vi "Write Sensor Attributes.vi"(9 "New":T1, 11 "Sensor DAO Class in":refnum<class "Sensor DAO Class.lvclass">) -> (3 "Sensor DAO Class out":refnum<class "Sensor DAO Class.lvclass">)   [LabVIEW 2013]
uses:
  Sensor DAO Class.lvclass
  XControls/Sensor Metadata.ctl
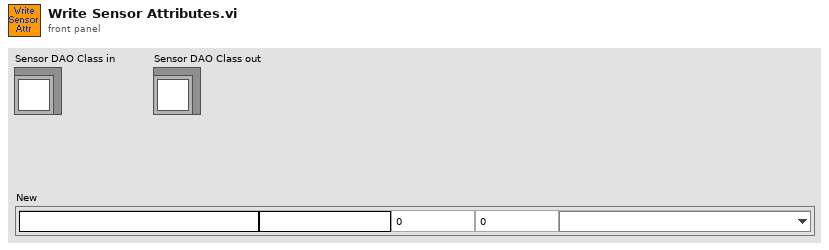
[diagram p1: front panel]
types:
  T1 = typedef "Sensor Metadata.ctl" = cluster{"Name":string, "Units":string, "Multiplier":dbl, "Excitation":u16, "Sensitivity":dbl}
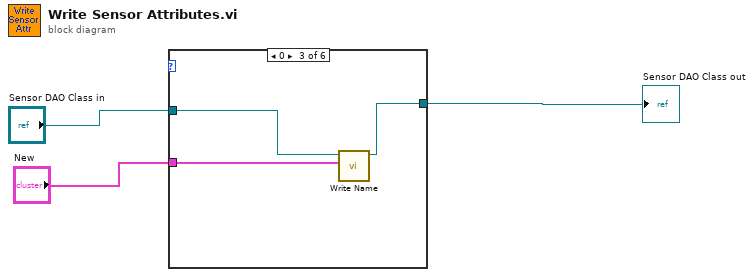
[diagram p0: block diagram]
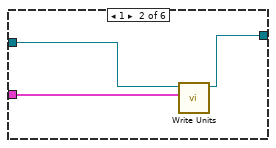
[diagram p3: hidden frame]
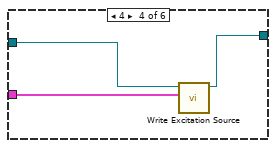
[diagram p4: hidden frame]
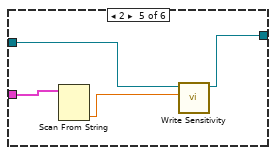
[diagram p5: hidden frame]
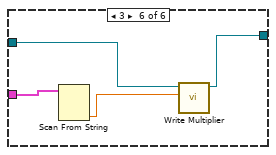
[diagram p6: hidden frame]
diagram:
  n1 = case shown="0" w1 {
    tunnel: "New" -> [_ w8 w11 w14 w18 w22]
    tunnel: "Sensor DAO Class in" -> [w5 w7 w10 w13 w17 w21]
    tunnel: [w5 w6 w9 w12 w16 w20] -> w4
    frame -1, Default {
    }
    frame 1 {
      n2 = call "Write Units.vi"("Units"=w8, "Sensor DAO Class in"=w7) -> ("Sensor DAO Class out"=w6:refnum<class "Sensor DAO Class.lvclass">)  [unwired: 8 in, 1 out]
    }
    frame 0 {
      n3 = call "Write Name.vi"("Name"=w11, "Sensor DAO Class in"=w10) -> ("Sensor DAO Class out"=w9:refnum<class "Sensor DAO Class.lvclass">)  [unwired: 8 in, 1 out]
    }
    frame 4 {
      n4 = call "Write Excitation Source.vi"("Excitation Source"=w14, "Sensor DAO Class in"=w13) -> ("Sensor DAO Class out"=w12:refnum<class "Sensor DAO Class.lvclass">)  [unwired: 8 in, 1 out]
    }
    frame 2 {
      n5 = Scan From String(input string=w18) -> (output 1=w15:dbl)  [unwired: 4 in, 3 out]
      n6 = call "Write Sensitivity.vi"("Sensitivity"=w15, "Sensor DAO Class in"=w17) -> ("Sensor DAO Class out"=w16:refnum<class "Sensor DAO Class.lvclass">)  [unwired: 8 in, 1 out]
    }
    frame 3 {
      n7 = Scan From String(input string=w22) -> (output 1=w19:dbl)  [unwired: 4 in, 3 out]
      n8 = call "Write Multiplier.vi"("Multiplier"=w19, "Sensor DAO Class in"=w21) -> ("Sensor DAO Class out"=w20:refnum<class "Sensor DAO Class.lvclass">)  [unwired: 8 in, 1 out]
    }
  }
  "Sensor DAO Class out" <- w4
